vi "InitPmuImpairParams.vi"(8 "ErrorArray In":errorcluster[](array[cluster])) -> (0 "ErrorArray Out":errorcluster[](array[cluster]))   [LabVIEW 2017, in "Framework.lvlib"]
uses:
  Framework.lvlib
  TypeDefs/clInitParams.ctl
  <vilib>/Utility/error.llb/Error Cluster From Error Code.vi
  <vilib>/ErrorRing/Error Ring.xnode
  <vilib>/Utility/config.llb/NI_LVConfig.lvlib
  <userlib>/NIST/NISTErrorLib/NISTErrorLib.lvlib
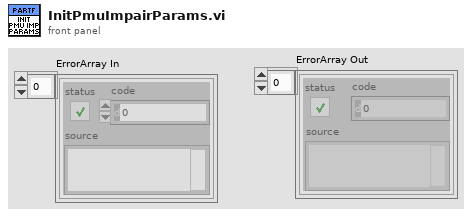
[diagram p1: front panel]
types:
  T1 = typedef "Framework.lvlib/clFrontPanelControlRefs.ctl" = cluster{"TestFilePathRef":refnum<vi>, "BusNumberRef":refnum<vi>, "NumberOfBusesRef":refnum<vi>, "EvtTypeRef":refnum<vi>, "EvtParamsRef":refnum<vi>, "EvtConfigRef":refnum<vi>, "StartTimeRef":refnum<vi>, "EndTimeRef":refnum<vi>, "PmuImpairTypeRef":refnum<vi>, "PmuImpairParamsRef":refnum<vi>, "NetImpairParamsRef":refnum<vi>, "FlagImpairTypeRef":refnum<vi>, "FlagImpairParamsRef":refnum<vi>, "NetImpairTypeRef":refnum<vi>, "OutputFileType":refnum<vi>, "PmuImpairConfigRef":refnum<vi>, "AppTypeRef":refnum<vi>, "ScriptPathRef":refnum<vi>, "ShowPanels?":refnum<vi>}
  T2 = typedef "Framework.lvlib/clInitParams.ctl" = cluster{"RowHdrs":string[], "ColHdrs":string[], "DefaultParams":string[][]}
  T3 = typedef "Framework.lvlib/clFrameworkData.ctl" = cluster{"EvtINIFilePaths":path[], "BusClassInstances":refnum<class "Bus.lvclass">[], "PmuImpairINIFilePaths":path[], "FlagImpairINIFilePaths":path[], "NetImpairINIFilePaths":path[], "OutputToFileINIFilePaths":path[], "AppINIFilePaths":path[], "AppModuleID":i32, "OutputToFileID":i32}
  T4 = typedef "NI_LVConfig.lvlib/Config Data RefNum.ctl" = refnum<k1>
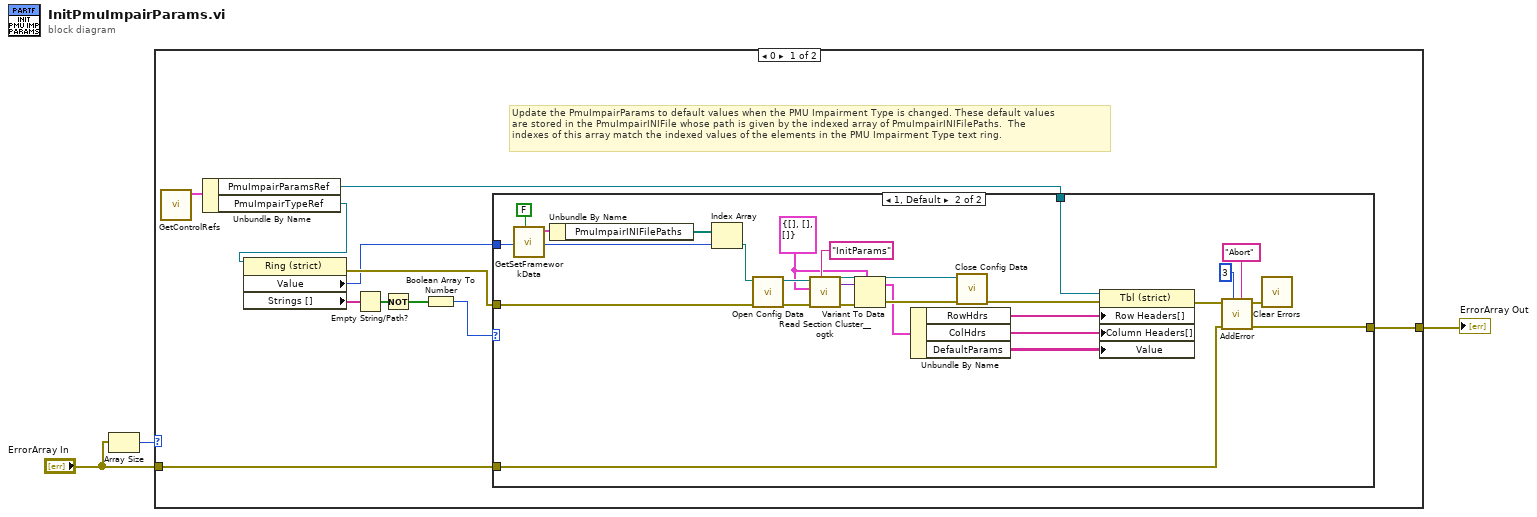
[diagram p0: block diagram]
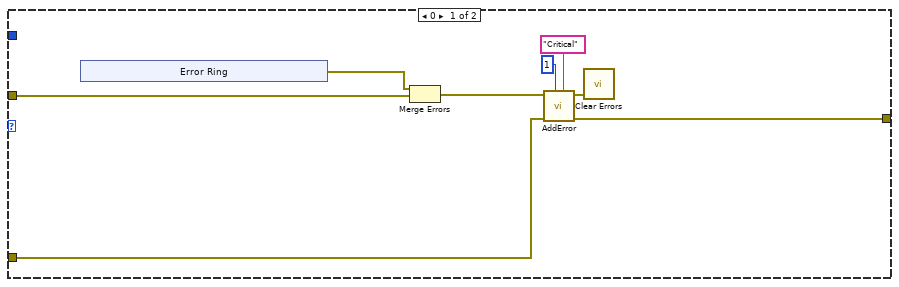
[diagram p2: hidden frame]
diagram:
  n1 = Array Size(array="ErrorArray In") -> (size(s)=w3:i32)
  n2 = case shown="0" w3 {
    tunnel: "ErrorArray In" -> [w9 w54]
    tunnel: [w8 w54] -> w1
    frame 0 {
      # "Update the PmuImpairParams to default values when the PMU Impairment Type is changed. These default values\nare stored in the PmuImpairINIFile whose path is given by the indexed array of PmuImpairINIFilePaths.  The \nindexes of this array match the indexed values of the elements in the PMU Impairment Type text ring."
      n3 = call "GetControlRefs.vi"() -> ("clControlRefs Out"=w4:T1)  [unwired: 11 in]
      n4 = Unbundle By Name(w4) -> ("PmuImpairParamsRef"=w11:refnum<vi>, "PmuImpairTypeRef"=w12:refnum<vi>)
      n5 = property class="Ring (strict)"(reference=w12) -> (error out=w14:errorcluster, "Value"=w13:u16, "Strings []"=w10:string[])  [unwired: 1 in, 1 out]
      n6 = Empty String/Path?(string/path=w10) -> (empty?=w7:bool[])
      n7 = Not(x=w7) -> (.not. x?=w5:bool[])
      n8 = Boolean Array To Number(Boolean array=w5) -> (number=w6:u32)
      n9 = case shown="1, Default" w6 {
        tunnel: w14 -> [w21 w39]
        tunnel: w13 -> [_ w38]
        tunnel: w11 -> [_ w31]
        tunnel: w9 -> [w16 w33]
        tunnel: [w15 w34] -> w8
        frame 0 {
          n10 = xnode "Error Ring"() -> ("error out"=w22:errorcluster)
          n11 = Merge Errors(w22, w21) -> (w17:errorcluster)
          n12 = call <userlib>:"AddError.vi"("Severity"="Critical" ("String"), "Priority"=u8 1, "ErrorArray"=w16, "error in (no error)"=w17) -> ("ErrorArray"=w15:errorcluster[], "error out"=w20:errorcluster)  [unwired: 6 in]
          n13 = call <vilib>:"Clear Errors.vi"("error in (no error)"=w20) -> ()  [unwired: 5 in, 2 out]
        }
        frame 1, Default {
          w28 = T2 {"RowHdrs"=[], "ColHdrs"=[], "DefaultParams"=[]} ("InitParams")
          n14 = call "GetSetFrameworkData.vi"("Set (F)"=FALSE ("Set/Get")) -> ("clFrameworkData Out"=w46:T3)  [unwired: 10 in]
          n15 = Unbundle By Name(w46) -> ("PmuImpairINIFilePaths"=w53:path[])
          n16 = Index Array(array=w53, index=w38) -> (element=w52:path)
          n17 = call <vilib>:"Open Config Data.vi"("error in (no error)"=w39, "configuration file path"=w52) -> ("error out"=w51:errorcluster, "refnum"=w50:T4)  [unwired: 7 in, 1 out]
          n18 = call <userlib>:"Read Section Cluster__ogtk.vi"("section (optional)"="InitParams", "error in (no error)"=w51, "Section Formatted Cluster Type"=w28, "refnum"=w50) -> ("error out"=w48:errorcluster, "Section Formatted Cluster"=w47:variant, "dup refnum"=w40:T4)  [unwired: 3 in, 2 out]
          n19 = Variant To Data(error in=w48, type=w28, Variant=w47) -> (data=w30:T2, error out=w41:errorcluster)
          n20 = Unbundle By Name(w30) -> ("RowHdrs"=w43:string[], "ColHdrs"=w44:string[], "DefaultParams"=w29:string[][])
          n21 = call <vilib>:"Close Config Data.vi"("error in (no error)"=w41, "refnum"=w40) -> ("error out"=w42:errorcluster)  [unwired: 8 in, 1 out]
          n22 = property on="Property Node" class="Tbl (strict)"(reference=w31, error in=w42, "Row Headers[]"=w43, "Column Headers[]"=w44, "Value"=w29) -> (error out=w32:errorcluster)  [unwired: 1 out]
          n23 = call <userlib>:"AddError.vi"("Severity"="Abort" ("String"), "Priority"=u8 3, "ErrorArray"=w33, "error in (no error)"=w32) -> ("ErrorArray"=w34:errorcluster[], "error out"=w35:errorcluster)  [unwired: 6 in]
          n24 = call <vilib>:"Clear Errors.vi"("error in (no error)"=w35) -> ()  [unwired: 5 in, 2 out]
        }
      }
    }
    frame 1, Default {
    }
  }
  "ErrorArray Out" <- w1
